vi "GetCurrentIndex.vi"(8 "Error In":errorcluster, 11 "reference in":refnum<class "Recipe.lvclass">) -> (0 "Error Out":errorcluster, 2 "Current Index":u64, 3 "reference out":refnum<class "Recipe.lvclass">)   [LabVIEW 2021, in "Recipe.lvclass"]
uses:
  Recipe.lvclass
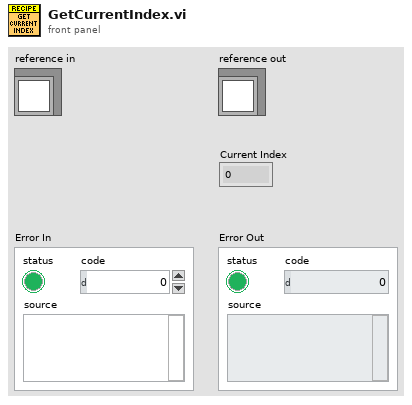
[diagram p1: front panel]
types:
  T1 = typedef "Recipe.lvclass/ObjectAttributes.ctl" = cluster{"Steps":refnum<class "Recipe Step.lvclass">[], "Current Info":cluster{"Current Index":u64}}
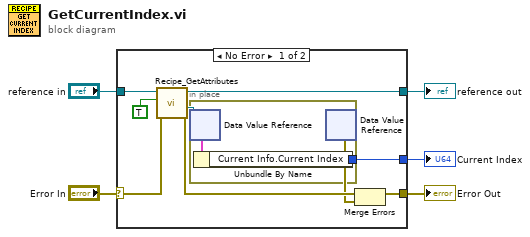
[diagram p0: block diagram]
diagram:
  n1 = case shown="No Error" "Error In" {
    selector: "Error In" -> [w14 w18]
    tunnel: [w12 w18] -> w4
    tunnel: [w9 w17] -> w2
    tunnel: "reference in" -> [w10 w17]
    tunnel: [w6 _] -> w1
    frame No Error {
      n2 = call "Recipe_GetAttributes.vi"("Error In"=w14, "OnlyGetDvrReference(False)"=TRUE, "reference in"=w10) -> ("Error Out"=w13:errorcluster, "DataRef"=w7:refnum<data-value>, "reference out"=w9:refnum<class "Recipe.lvclass">)  [unwired: 5 in, 1 out]
      n3 = in-place {
        in-place-border: [w16] -> w6
        n4 = in-place-dvr #1(w7) -> (w15:T1)  [unwired: 1 out]
        n5 = Unbundle By Name(w15) -> ("Current Info.Current Index"=w16:u64)
        n6 = in-place-dvr #1() -> (w11:errorcluster)  [unwired: 1 in, 1 out]
      }
      n7 = Merge Errors(w13, w11) -> (w12:errorcluster)
    }
    frame Error {
    }
  }
  "Error Out" <- w4
  "reference out" <- w2
  "Current Index" <- w1
